vi "Create ToolStripSeperator.vi"(8 "error in (no error)":errorcluster caption="错误输入（无错误）", 11 "StatusStripClass 输入":refnum<class "StatusStripClass.lvclass"> caption="DNL_LabVIEW Object in") -> (0 "error out":errorcluster caption="错误输出", 3 "StatusStripClass 输出":refnum<class "StatusStripClass.lvclass"> caption="DNL_LabVIEW Object out")   [LabVIEW 2013, in "StatusStripClass.lvclass"]
uses:
  StatusStripClass.lvclass
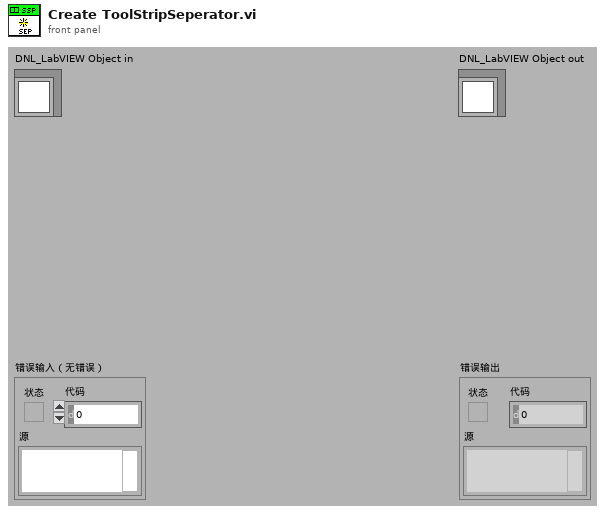
[diagram p1: front panel]
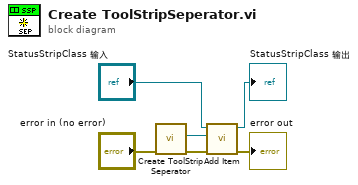
[diagram p0: block diagram]
diagram:
  n1 = call "Create ToolStrip Seperator.vi"("error in (no error)"="error in (no error)") -> ("error out"=w4:errorcluster, "ItemRef"=w5:refnum<k24>)  [unwired: 8 in, 1 out]
  n2 = call "Add Item.vi"("error in (no error)"=w4, "ItemRef"=w5, "StatusStripClass 输入"="StatusStripClass 输入") -> ("error out"=→"error out":errorcluster, "StatusStripClass 输出"=→"StatusStripClass 输出":refnum<class "StatusStripClass.lvclass">)  [unwired: 7 in]
